vi "map_diag_stiffback.vi"() -> ()   [LabVIEW 2015]
panel:
  in  "Done ?":bool
  out "Mapping DX ext":string
  out "Mapping SX ext":string
  out "Mapping DX int":string
  out "Mapping SX int":string
  in  "z inizio":bool
  in  "x piastra":bool
  in  "z piastra":bool
  in  "Done":bool
  in  "y inizio":bool
  in  "Positioning Done":bool
  in  "x inizio":bool
  in  "y inizio":bool
  in  "Positioning Done":bool
  in  "y inizio":bool
  in  "Positioning Done":bool
  in  "KILL":bool
  in  "PAUSE":bool
  in  "RESUME":bool
  in  "QUIT":bool
  in  "Positioning Done":bool
  in  "y inizio":bool
  in  "x inizio":bool
  in  "End":bool
  in  "zero z - end":bool
  in  "zero x - end":bool
  in  "zero y - end":bool
  out "output":string
  out "command":string
  in  "zero done":bool
  in  "zero z":bool
  in  "zero x":bool
  in  "zero y":bool
  # "Posiziono in zero"
  # "Comandi di emergenza"
  # "Vado al punto di \nazzeramento"
  # "Vado al punto di partenza\nDiagonale Left Internal"
  # "Vado al punto di partenza\nDiagonale Right Internal"
  # "Vado al punto di partenza\nDiagonale Left External"
  # "Vado al punto di partenza\nDiagonale Right External"
  # "Ritorno a zero"
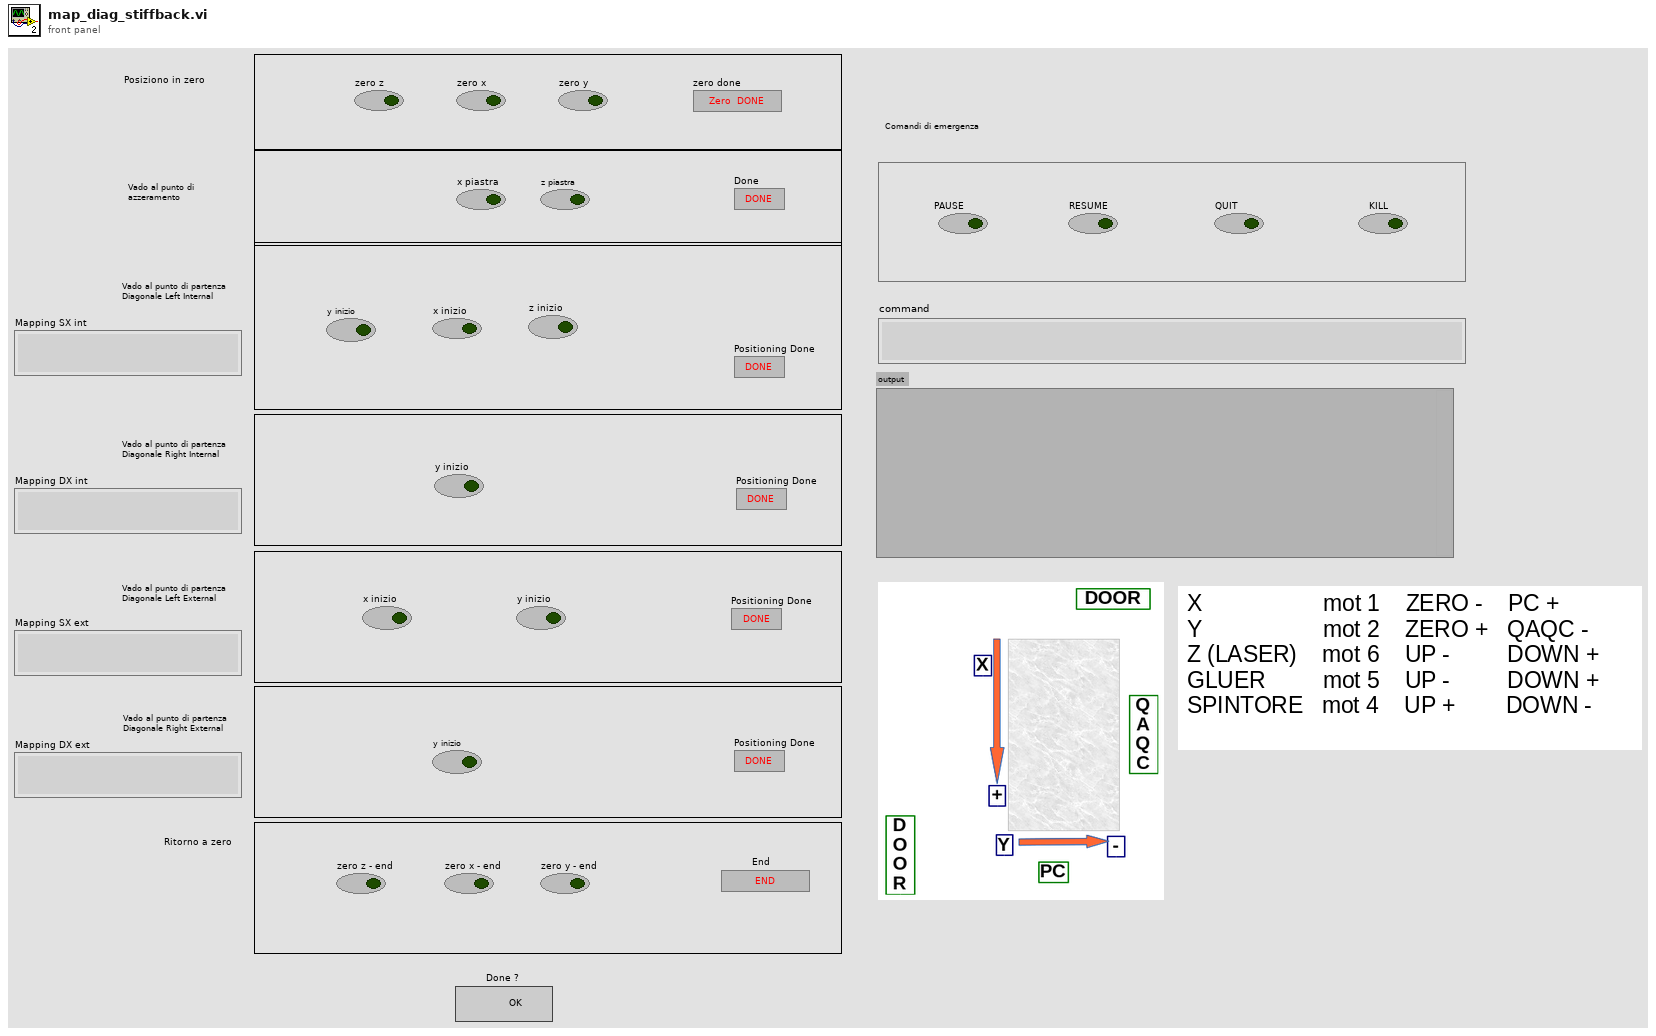
[diagram p1: front panel]
types:
  T1 = enum16{"open", "replace", "create", "open or create", "replace or create", "replace or create with confirmation"}
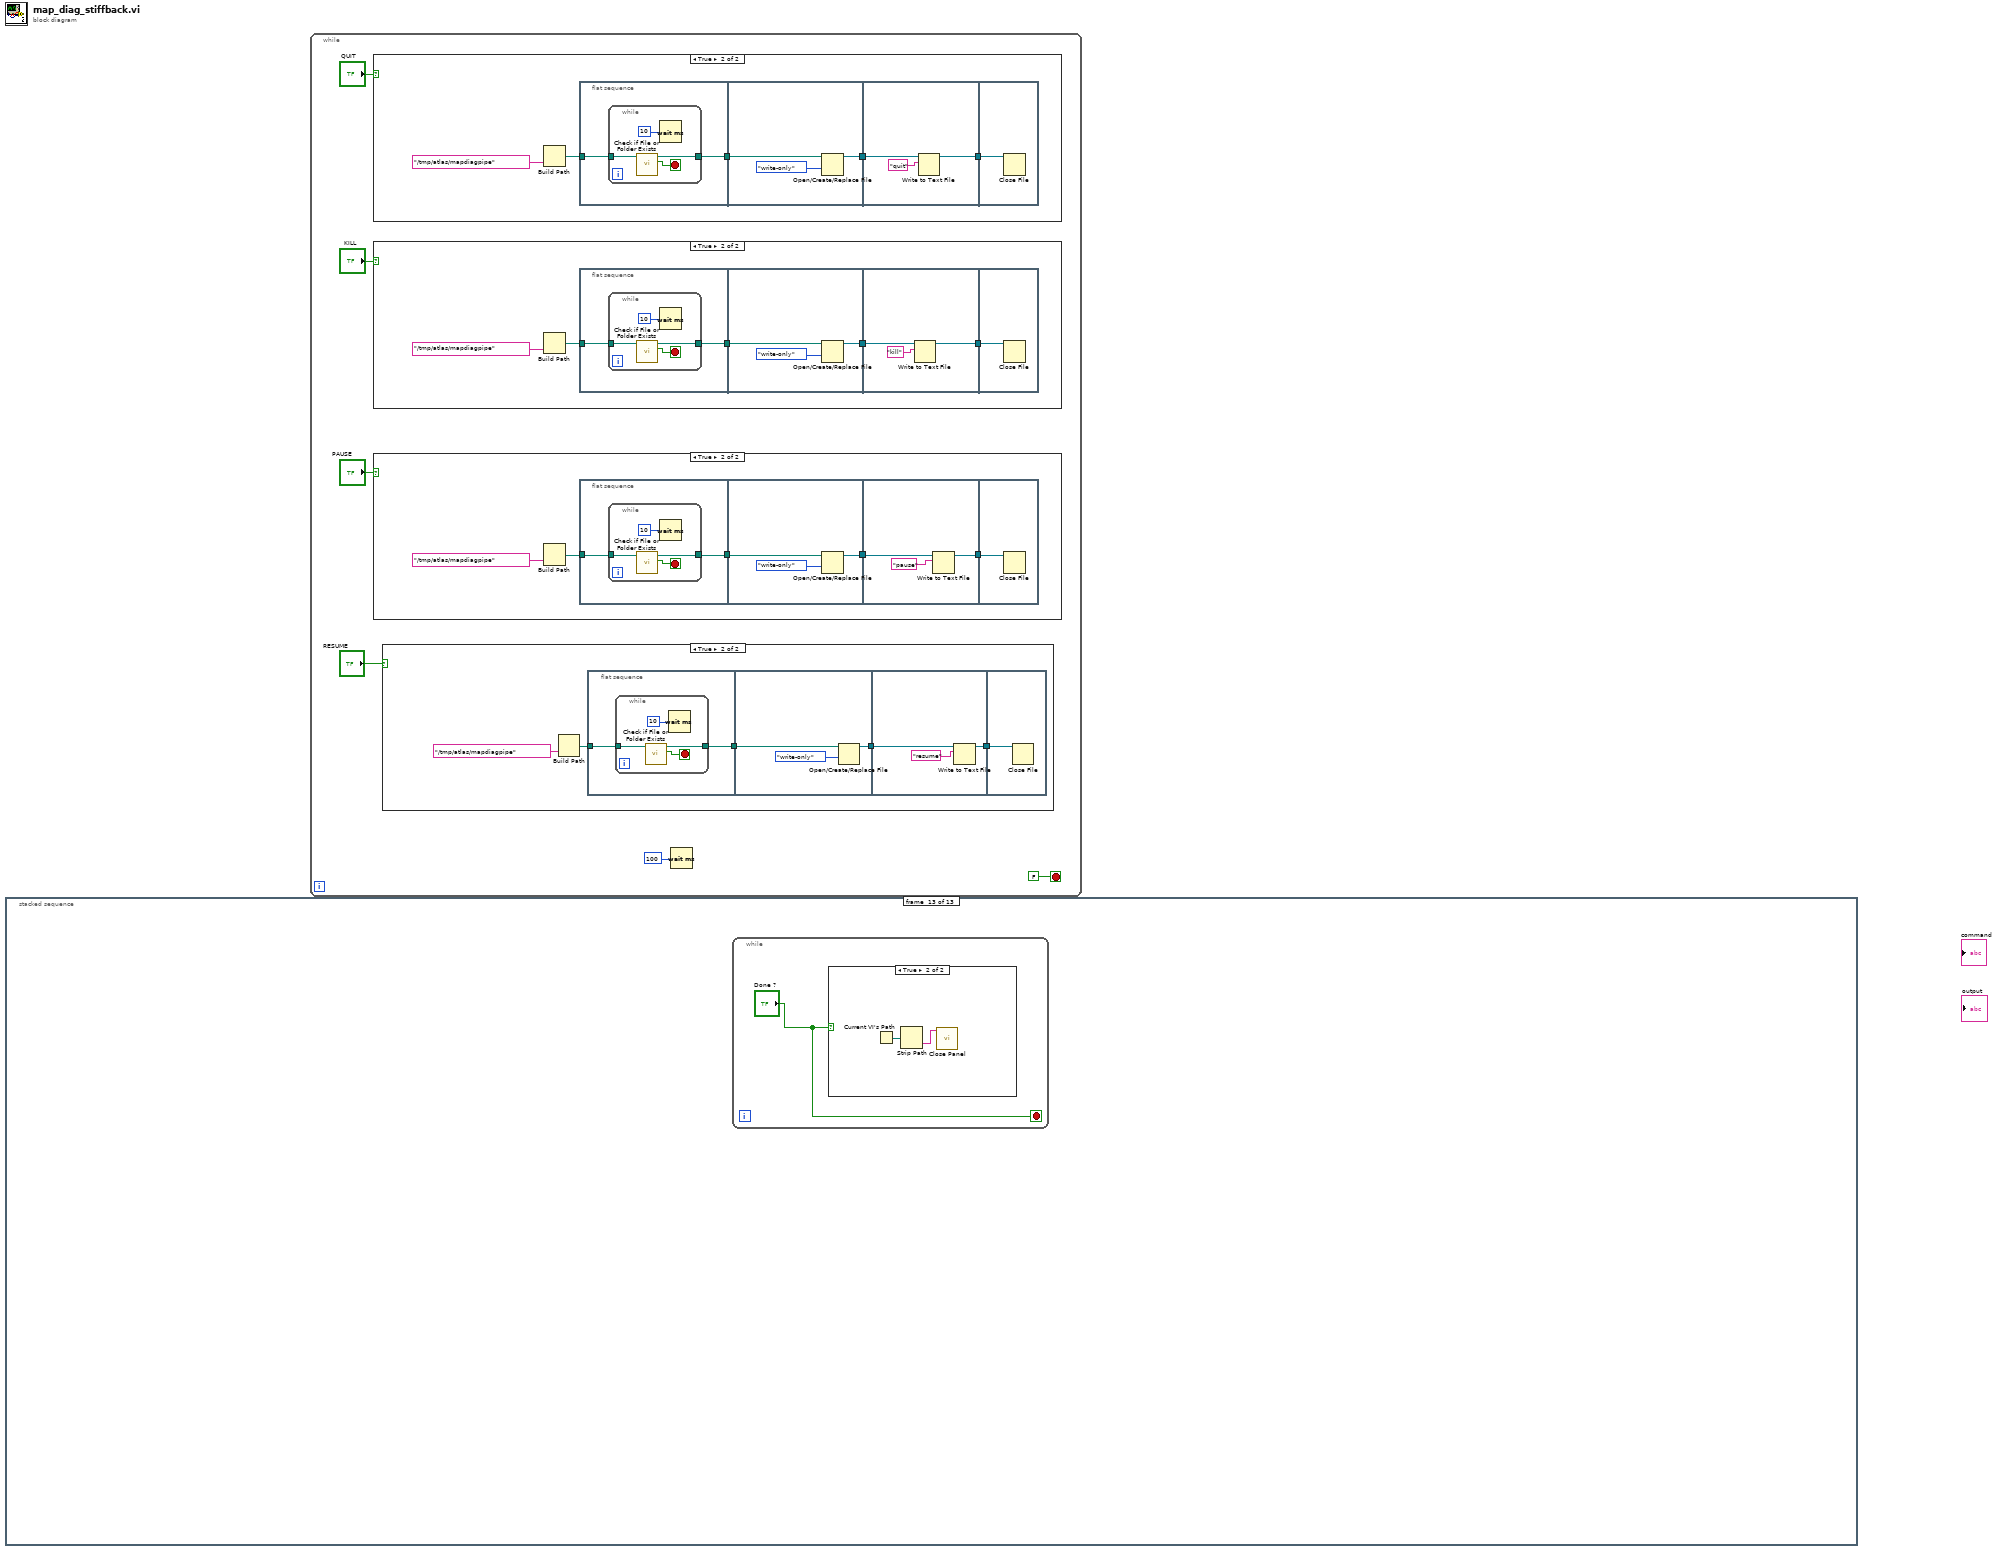
[diagram p0: block diagram]
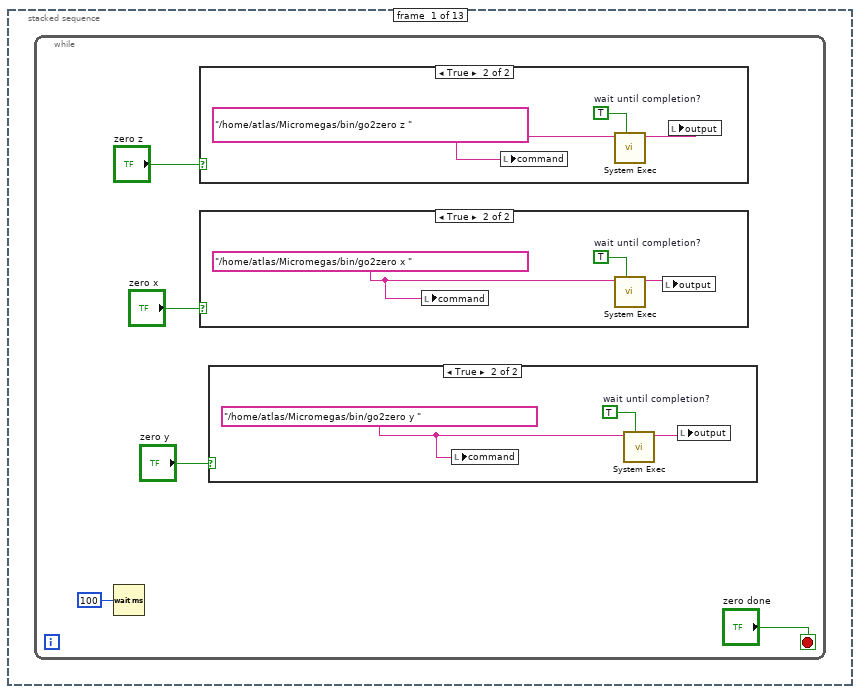
[diagram p6: hidden frame]
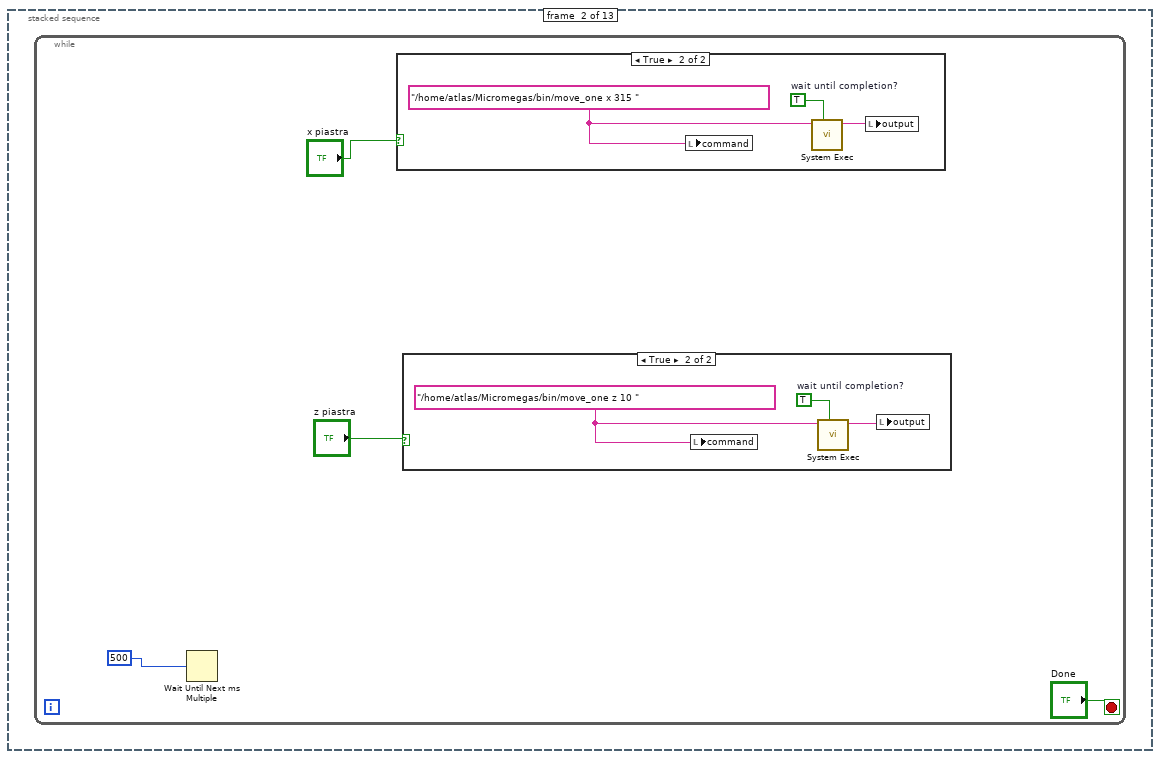
[diagram p10: hidden frame]
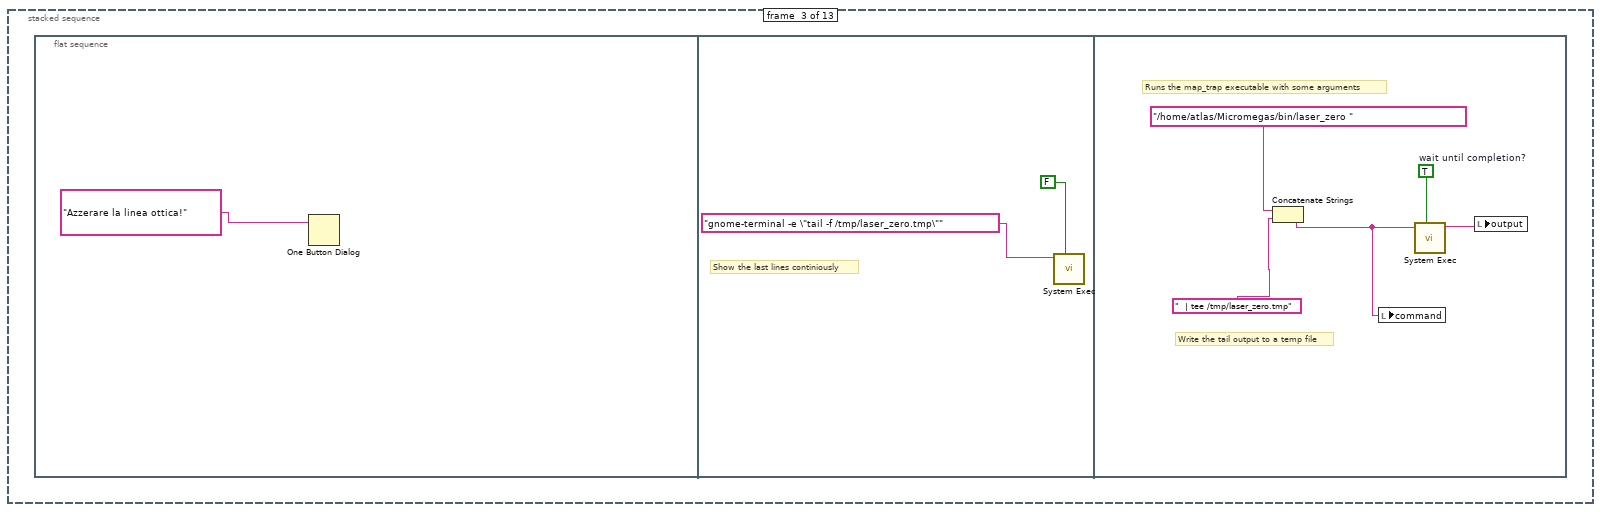
[diagram p13: hidden frame]
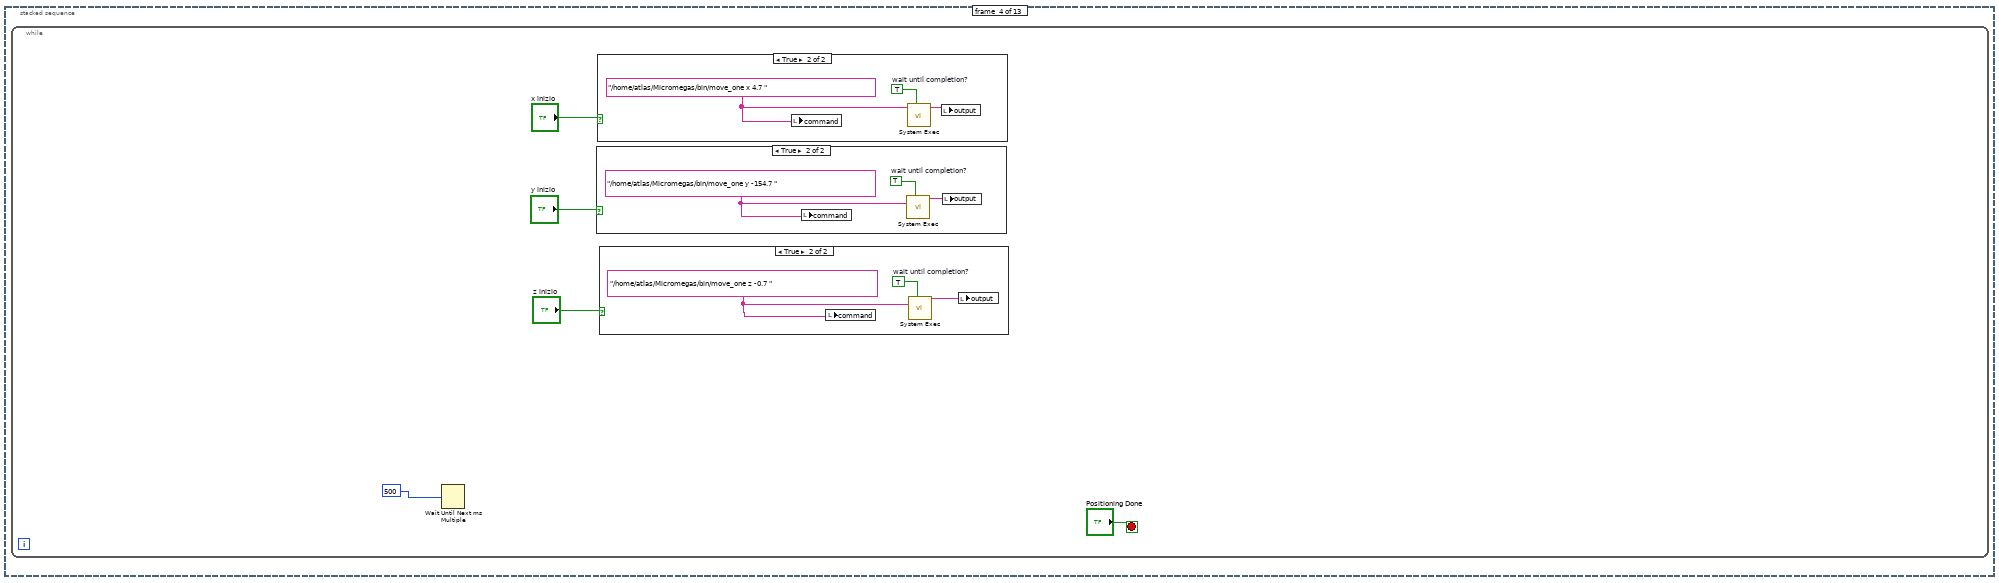
[diagram p14: hidden frame]
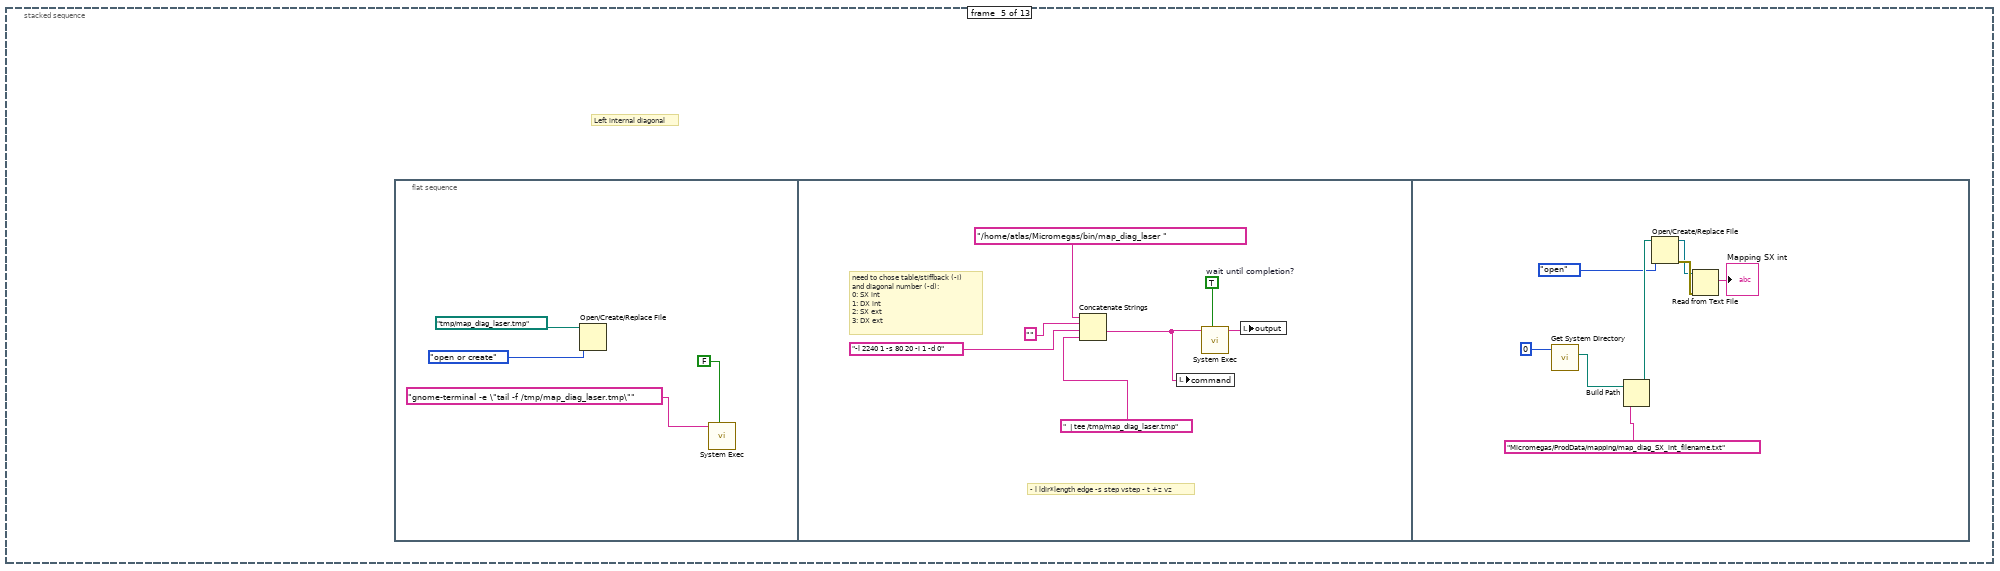
[diagram p18: hidden frame]
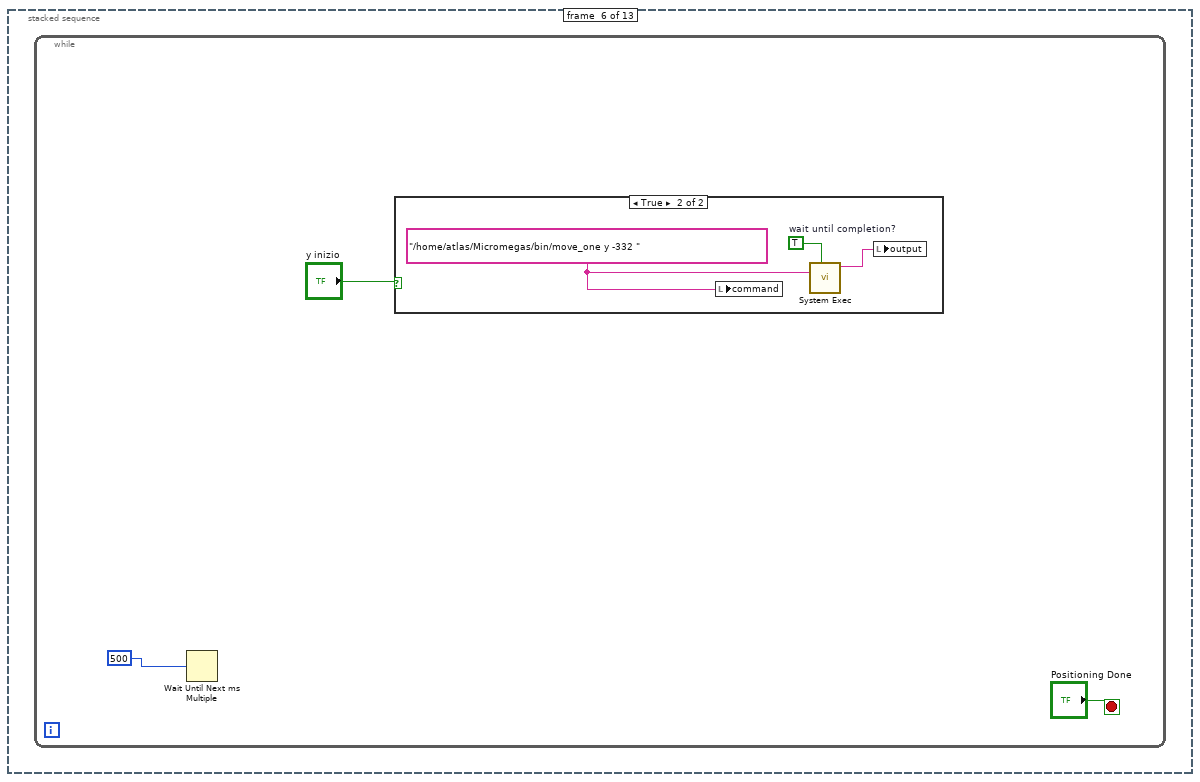
[diagram p19: hidden frame]
diagram:
  n1 = stacked-sequence {
    frame #0 {
      n2 = while {
        stop <- "zero done" stop-if-true
        n3 = Wait (ms)(milliseconds to wait=u32 100) -> ()  [unwired: 1 out]
        n4 = case shown="True" "zero z" {
          frame False {
          }
          frame True {
            w13 = "/home/atlas/Micromegas/bin/go2zero z " ("string")
            w14 = TRUE  # wait until completion?
            n5 = local write "command"(w13) -> ()
            n6 = call <vilib>:"System Exec.vi"("wait until completion? (T)"=w14, "command line"=w13) -> ("standard output"=w12:string)  [unwired: 6 in, 3 out]
            n7 = local write "output"(w12) -> ()
          }
        }
        n8 = case shown="True" "zero x" {
          frame False {
          }
          frame True {
            w10 = "/home/atlas/Micromegas/bin/go2zero x " ("string")
            w11 = TRUE  # wait until completion?
            n9 = local write "command"(w10) -> ()
            n10 = call <vilib>:"System Exec.vi"("wait until completion? (T)"=w11, "command line"=w10) -> ("standard output"=w9:string)  [unwired: 6 in, 3 out]
            n11 = local write "output"(w9) -> ()
          }
        }
        n12 = case shown="True" "zero y" {
          frame False {
          }
          frame True {
            w7 = "/home/atlas/Micromegas/bin/go2zero y " ("string")
            w8 = TRUE  # wait until completion?
            n13 = local write "command"(w7) -> ()
            n14 = call <vilib>:"System Exec.vi"("wait until completion? (T)"=w8, "command line"=w7) -> ("standard output"=w6:string)  [unwired: 6 in, 3 out]
            n15 = local write "output"(w6) -> ()
          }
        }
      }
    }
    frame #1 {
      n16 = while {
        stop <- "Done" stop-if-true
        n17 = Wait Until Next ms Multiple(millisecond multiple=u32 500 ("millisecond timer value")) -> ()  [unwired: 1 out]
        n18 = case shown="True" "x piastra" {
          frame False {
          }
          frame True {
            w22 = "/home/atlas/Micromegas/bin/move_one x 315 " ("string")
            w24 = TRUE  # wait until completion?
            n19 = local write "command"(w22) -> ()
            n20 = call <vilib>:"System Exec.vi"("wait until completion? (T)"=w24, "command line"=w22) -> ("standard output"=w23:string)  [unwired: 6 in, 3 out]
            n21 = local write "output"(w23) -> ()
          }
        }
        n22 = case shown="True" "z piastra" {
          frame False {
          }
          frame True {
            w20 = "/home/atlas/Micromegas/bin/move_one z 10 " ("string")
            w21 = TRUE  # wait until completion?
            n23 = local write "command"(w20) -> ()
            n24 = call <vilib>:"System Exec.vi"("wait until completion? (T)"=w21, "command line"=w20) -> ("standard output"=w19:string)  [unwired: 6 in, 3 out]
            n25 = local write "output"(w19) -> ()
          }
        }
      }
    }
    frame #2 {
      n26 = flat-sequence {
        frame #0 {
          n27 = One Button Dialog(message="Azzerare la linea ottica!") -> ()  [unwired: 1 in, 1 out]
        }
        frame #1 {
          # "Show the last lines continiously"
          n28 = call <vilib>:"System Exec.vi"("wait until completion? (T)"=FALSE, "command line"="gnome-terminal -e \"tail -f /tmp/laser_zero.tmp\"") -> ()  [unwired: 6 in, 4 out]
        }
        frame #2 {
          w32 = TRUE  # wait until completion?
          # "Write the tail output to a temp file"
          # "Runs the map_trap executable with some arguments"
          n29 = Concatenate Strings("/home/atlas/Micromegas/bin/laser_zero " ("string"), "  | tee /tmp/laser_zero.tmp" ("string")) -> (w28:string)
          n30 = local write "command"(w28) -> ()
          n31 = call <vilib>:"System Exec.vi"("wait until completion? (T)"=w32, "command line"=w28) -> ("standard output"=w29:string)  [unwired: 6 in, 3 out]
          n32 = local write "output"(w29) -> ()
        }
      }
    }
    frame #3 {
      n33 = while {
        stop <- "Positioning Done" stop-if-true
        n34 = Wait Until Next ms Multiple(millisecond multiple=u32 500 ("millisecond timer value")) -> ()  [unwired: 1 out]
        n35 = case shown="True" "y inizio" {
          frame False {
          }
          frame True {
            w41 = "/home/atlas/Micromegas/bin/move_one y -154.7 " ("string")
            w43 = TRUE  # wait until completion?
            n36 = local write "command"(w41) -> ()
            n37 = call <vilib>:"System Exec.vi"("wait until completion? (T)"=w43, "command line"=w41) -> ("standard output"=w42:string)  [unwired: 6 in, 3 out]
            n38 = local write "output"(w42) -> ()
          }
        }
        n39 = case shown="True" "x inizio" {
          frame False {
          }
          frame True {
            w44 = "/home/atlas/Micromegas/bin/move_one x 4.7 " ("string")
            w46 = TRUE  # wait until completion?
            n40 = local write "command"(w44) -> ()
            n41 = call <vilib>:"System Exec.vi"("wait until completion? (T)"=w46, "command line"=w44) -> ("standard output"=w45:string)  [unwired: 6 in, 3 out]
            n42 = local write "output"(w45) -> ()
          }
        }
        n43 = case shown="True" "z inizio" {
          frame False {
          }
          frame True {
            w38 = "/home/atlas/Micromegas/bin/move_one z -0.7 " ("string")
            w40 = TRUE  # wait until completion?
            n44 = local write "command"(w38) -> ()
            n45 = call <vilib>:"System Exec.vi"("wait until completion? (T)"=w40, "command line"=w38) -> ("standard output"=w39:string)  [unwired: 6 in, 3 out]
            n46 = local write "output"(w39) -> ()
          }
        }
      }
    }
    frame #4 {
      # "Left internal diagonal"
      n47 = flat-sequence {
        frame #0 {
          n48 = Open/Create/Replace File(file path (use dialog)=path "/tmp/map_diag_laser.tmp", operation (0:open)=T1."open or create") -> ()  [unwired: 4 in, 3 out]
          n49 = call <vilib>:"System Exec.vi"("wait until completion? (T)"=FALSE, "command line"="gnome-terminal -e \"tail -f /tmp/map_diag_laser.tmp\"") -> ()  [unwired: 6 in, 4 out]
        }
        frame #1 {
          w57 = TRUE  # wait until completion?
          # "need to chose table/stiffback (-i)\nand diagonal number (-d):\n0: SX int\n1: DX int\n2: SX ext\n3: DX ext"
          # "- l ldir*length edge -s step vstep - t +z vz"
          n50 = Concatenate Strings("/home/atlas/Micromegas/bin/map_diag_laser " ("string"), "" ("string"), "-l 2240 1 -s 80 20 -i 1 -d 0" ("string"), "  | tee /tmp/map_diag_laser.tmp" ("string")) -> (w54:string)
          n51 = local write "command"(w54) -> ()
          n52 = call <vilib>:"System Exec.vi"("wait until completion? (T)"=w57, "command line"=w54) -> ("standard output"=w55:string)  [unwired: 6 in, 3 out]
          n53 = local write "output"(w55) -> ()
        }
        frame #2 {
          n54 = call <vilib>:"Get System Directory.vi"("system directory type"=0) -> ("system directory"=w64:path)  [unwired: 10 in]
          n55 = Build Path(base path=w64, name or relative path="Micromegas/ProdData/mapping/map_diag_SX_int_filename.txt") -> (appended path=w65:path)
          n56 = Open/Create/Replace File(file path (use dialog)=w65, operation (0:open)=T1."open") -> (refnum out=w59:refnum<file>, error out=w60:errorcluster)  [unwired: 4 in, 1 out]
          n57 = Read from Text File(file (use dialog)=w59, error in=w60) -> (text=→"Mapping SX int":string)  [unwired: 2 in, 3 out]
        }
      }
    }
    frame #5 {
      n58 = while {
        stop <- "Positioning Done" stop-if-true
        n59 = Wait Until Next ms Multiple(millisecond multiple=u32 500 ("millisecond timer value")) -> ()  [unwired: 1 out]
        n60 = case shown="True" "y inizio" {
          frame False {
          }
          frame True {
            w69 = "/home/atlas/Micromegas/bin/move_one y -332 " ("string")
            w71 = TRUE  # wait until completion?
            n61 = local write "command"(w69) -> ()
            n62 = call <vilib>:"System Exec.vi"("wait until completion? (T)"=w71, "command line"=w69) -> ("standard output"=w70:string)  [unwired: 6 in, 3 out]
            n63 = local write "output"(w70) -> ()
          }
        }
      }
    }
    frame #6 {
      n64 = flat-sequence {
        frame #0 {
          w78 = TRUE  # wait until completion?
          # "need to chose table/stiffback (-i)\nand diagonal number (-d):\n0: SX int\n1: DX int\n2: SX ext\n3: DX ext"
          # "Right internal diagonal"
          # "- l ldir*length edge -s step vstep - t +z vz"
          n65 = Concatenate Strings("/home/atlas/Micromegas/bin/map_diag_laser " ("string"), "" ("string"), "-l -2240 0 -s 80 20 -i 1 -d 1" ("string"), "  | tee /tmp/map_diag_laser.tmp" ("string")) -> (w72:string)
          n66 = call <vilib>:"System Exec.vi"("wait until completion? (T)"=w78, "command line"=w72) -> ("standard output"=w73:string)  [unwired: 6 in, 3 out]
          n67 = local write "command"(w72) -> ()
          n68 = local write "output"(w73) -> ()
        }
        frame #1 {
          n69 = call <vilib>:"Get System Directory.vi"("system directory type"=0) -> ("system directory"=w85:path)  [unwired: 10 in]
          n70 = Build Path(base path=w85, name or relative path="Micromegas/ProdData/mapping/map_diag_DX_int_filename.txt") -> (appended path=w86:path)
          n71 = Open/Create/Replace File(file path (use dialog)=w86, operation (0:open)=T1."open") -> (refnum out=w80:refnum<file>, error out=w81:errorcluster)  [unwired: 4 in, 1 out]
          n72 = Read from Text File(file (use dialog)=w80, error in=w81) -> (text=→"Mapping DX int":string)  [unwired: 2 in, 3 out]
        }
      }
    }
    frame #7 {
      n73 = while {
        stop <- "Positioning Done" stop-if-true
        n74 = Wait Until Next ms Multiple(millisecond multiple=u32 500 ("millisecond timer value")) -> ()  [unwired: 1 out]
        n75 = case shown="True" "x inizio" {
          frame False {
          }
          frame True {
            w91 = "/home/atlas/Micromegas/bin/move_one x 11 " ("string")
            w93 = TRUE  # wait until completion?
            n76 = local write "command"(w91) -> ()
            n77 = call <vilib>:"System Exec.vi"("wait until completion? (T)"=w93, "command line"=w91) -> ("standard output"=w92:string)  [unwired: 6 in, 3 out]
            n78 = local write "output"(w92) -> ()
          }
        }
        n79 = case shown="True" "y inizio" {
          frame False {
          }
          frame True {
            w94 = "/home/atlas/Micromegas/bin/move_one y 1190 " ("string")
            w96 = TRUE  # wait until completion?
            n80 = local write "command"(w94) -> ()
            n81 = call <vilib>:"System Exec.vi"("wait until completion? (T)"=w96, "command line"=w94) -> ("standard output"=w95:string)  [unwired: 6 in, 3 out]
            n82 = local write "output"(w95) -> ()
          }
        }
      }
    }
    frame #8 {
      n83 = flat-sequence {
        frame #0 {
          w103 = TRUE  # wait until completion?
          # "need to chose table/stiffback (-i)\nand diagonal number (-d):\n0: SX int\n1: DX int\n2: SX ext\n3: DX ext"
          # "Left external diagonal"
          # "- l ldir*length edge -s step vstep - t +z vz"
          n84 = Concatenate Strings("/home/atlas/Micromegas/bin/map_diag_laser " ("string"), "" ("string"), "-l 2200 1 -s 110 20 -i 1 -d 2" ("string"), "  | tee /tmp/map_diag_laser.tmp" ("string")) -> (w97:string)
          n85 = call <vilib>:"System Exec.vi"("wait until completion? (T)"=w103, "command line"=w97) -> ("standard output"=w98:string)  [unwired: 6 in, 3 out]
          n86 = local write "command"(w97) -> ()
          n87 = local write "output"(w98) -> ()
        }
        frame #1 {
          n88 = call <vilib>:"Get System Directory.vi"("system directory type"=0) -> ("system directory"=w110:path)  [unwired: 10 in]
          n89 = Build Path(base path=w110, name or relative path="Micromegas/ProdData/mapping/map_diag_SX_ext_filename.txt") -> (appended path=w111:path)
          n90 = Open/Create/Replace File(file path (use dialog)=w111, operation (0:open)=T1."open") -> (refnum out=w105:refnum<file>, error out=w106:errorcluster)  [unwired: 4 in, 1 out]
          n91 = Read from Text File(file (use dialog)=w105, error in=w106) -> (text=→"Mapping SX ext":string)  [unwired: 2 in, 3 out]
        }
      }
    }
    frame #9 {
      n92 = while {
        stop <- "Positioning Done" stop-if-true
        n93 = Wait Until Next ms Multiple(millisecond multiple=u32 500 ("millisecond timer value")) -> ()  [unwired: 1 out]
        n94 = case shown="True" "y inizio" {
          frame False {
          }
          frame True {
            w115 = "/home/atlas/Micromegas/bin/move_one y -505 " ("string")
            w117 = TRUE  # wait until completion?
            n95 = local write "command"(w115) -> ()
            n96 = call <vilib>:"System Exec.vi"("wait until completion? (T)"=w117, "command line"=w115) -> ("standard output"=w116:string)  [unwired: 6 in, 3 out]
            n97 = local write "output"(w116) -> ()
          }
        }
      }
    }
    frame #10 {
      n98 = flat-sequence {
        frame #0 {
          w124 = TRUE  # wait until completion?
          # "need to chose table/stiffback (-i)\nand diagonal number (-d):\n0: SX int\n1: DX int\n2: SX ext\n3: DX ext"
          # "Right external diagonal"
          # "- l ldir*length edge -s step vstep - t +z vz"
          n99 = Concatenate Strings("/home/atlas/Micromegas/bin/map_diag_laser " ("string"), "" ("string"), "-l -2200 0 -s 110 20 -i 1 -d 3" ("string"), "  | tee /tmp/map_diag_laser.tmp" ("string")) -> (w118:string)
          n100 = call <vilib>:"System Exec.vi"("wait until completion? (T)"=w124, "command line"=w118) -> ("standard output"=w119:string)  [unwired: 6 in, 3 out]
          n101 = local write "command"(w118) -> ()
          n102 = local write "output"(w119) -> ()
        }
        frame #1 {
          n103 = call <vilib>:"Get System Directory.vi"("system directory type"=0) -> ("system directory"=w131:path)  [unwired: 10 in]
          n104 = Build Path(base path=w131, name or relative path="Micromegas/ProdData/mapping/map_diag_DX_ext_filename.txt") -> (appended path=w132:path)
          n105 = Open/Create/Replace File(file path (use dialog)=w132, operation (0:open)=T1."open") -> (refnum out=w126:refnum<file>, error out=w127:errorcluster)  [unwired: 4 in, 1 out]
          n106 = Read from Text File(file (use dialog)=w126, error in=w127) -> (text=→"Mapping DX ext":string)  [unwired: 2 in, 3 out]
        }
      }
    }
    frame #11 {
      n107 = while {
        stop <- "End" stop-if-true
        n108 = Wait (ms)(milliseconds to wait=u32 100) -> ()  [unwired: 1 out]
        n109 = case shown="True" "zero z - end" {
          frame False {
          }
          frame True {
            w145 = "/home/atlas/Micromegas/bin/go2zero z " ("string")
            w146 = TRUE  # wait until completion?
            n110 = local write "command"(w145) -> ()
            n111 = call <vilib>:"System Exec.vi"("wait until completion? (T)"=w146, "command line"=w145) -> ("standard output"=w144:string)  [unwired: 6 in, 3 out]
            n112 = local write "output"(w144) -> ()
          }
        }
        n113 = case shown="True" "zero x - end" {
          frame False {
          }
          frame True {
            w142 = "/home/atlas/Micromegas/bin/go2zero x " ("string")
            w143 = TRUE  # wait until completion?
            n114 = local write "command"(w142) -> ()
            n115 = call <vilib>:"System Exec.vi"("wait until completion? (T)"=w143, "command line"=w142) -> ("standard output"=w141:string)  [unwired: 6 in, 3 out]
            n116 = local write "output"(w141) -> ()
          }
        }
        n117 = case shown="True" "zero y - end" {
          frame False {
          }
          frame True {
            w139 = "/home/atlas/Micromegas/bin/go2zero y " ("string")
            w140 = TRUE  # wait until completion?
            n118 = local write "command"(w139) -> ()
            n119 = call <vilib>:"System Exec.vi"("wait until completion? (T)"=w140, "command line"=w139) -> ("standard output"=w138:string)  [unwired: 6 in, 3 out]
            n120 = local write "output"(w138) -> ()
          }
        }
      }
    }
    frame #12 {
      n121 = while {
        stop <- "Done ?" stop-if-true
        n122 = case shown="True" "Done ?" {
          frame False {
          }
          frame True {
            n123 = Current VI's Path() -> (path=w148:path)
            n124 = Strip Path(path=w148) -> (name=w149:string)  [unwired: 1 out]
            n125 = call <vilib>:"Close Panel.vi"("VI name"=w149) -> ()  [unwired: 10 in, 1 out]
          }
        }
      }
    }
  }
  n126 = while {
    stop <- FALSE stop-if-true
    n127 = case shown="True" "QUIT" {
      frame False {
      }
      frame True {
        n128 = Build Path(name or relative path="/tmp/atlas/mapdiagpipe" ("string")) -> (appended path=w210:path)  [unwired: 1 in]
        n129 = flat-sequence {
          tunnel: [w216] -> w214
          tunnel: w210 -> [w215]
          tunnel: w214 -> [w223]
          tunnel: [w221] -> w213
          tunnel: w213 -> [w226]
          tunnel: [w225] -> w212
          tunnel: w212 -> [w227]
          frame #0 {
            n130 = while {
              tunnel: [w218] -> w216
              tunnel: w215 -> [w217]
              stop <- w219 stop-if-true
              n131 = call <vilib>:"Check if File or Folder Exists.vi"("path"=w217) -> ("file or folder exists?"=w219:bool, "dup path"=w218:path)  [unwired: 8 in, 1 out]
              n132 = Wait (ms)(milliseconds to wait=u32 10) -> ()  [unwired: 1 out]
            }
          }
          frame #1 {
            n133 = Open/Create/Replace File(file path (use dialog)=w223, access (0:read/write)=enum16{"read/write", "read-only", "write-only"}."write-only") -> (refnum out=w221:refnum<file>)  [unwired: 4 in, 2 out]
          }
          frame #2 {
            n134 = Write to Text File(file (use dialog)=w226, text="quit") -> (refnum out=w225:refnum<file>)  [unwired: 2 in, 2 out]
          }
          frame #3 {
            n135 = Close File(refnum=w227) -> ()  [unwired: 1 in, 2 out]
          }
        }
      }
    }
    n136 = case shown="True" "KILL" {
      frame False {
      }
      frame True {
        n137 = Build Path(name or relative path="/tmp/atlas/mapdiagpipe" ("string")) -> (appended path=w174:path)  [unwired: 1 in]
        n138 = flat-sequence {
          tunnel: [w180] -> w178
          tunnel: w174 -> [w179]
          tunnel: w178 -> [w187]
          tunnel: [w185] -> w177
          tunnel: w177 -> [w190]
          tunnel: [w189] -> w176
          tunnel: w176 -> [w191]
          frame #0 {
            n139 = while {
              tunnel: [w182] -> w180
              tunnel: w179 -> [w181]
              stop <- w183 stop-if-true
              n140 = call <vilib>:"Check if File or Folder Exists.vi"("path"=w181) -> ("file or folder exists?"=w183:bool, "dup path"=w182:path)  [unwired: 8 in, 1 out]
              n141 = Wait (ms)(milliseconds to wait=u32 10) -> ()  [unwired: 1 out]
            }
          }
          frame #1 {
            n142 = Open/Create/Replace File(file path (use dialog)=w187, access (0:read/write)=enum16{"read/write", "read-only", "write-only"}."write-only") -> (refnum out=w185:refnum<file>)  [unwired: 4 in, 2 out]
          }
          frame #2 {
            n143 = Write to Text File(file (use dialog)=w190, text="kill") -> (refnum out=w189:refnum<file>)  [unwired: 2 in, 2 out]
          }
          frame #3 {
            n144 = Close File(refnum=w191) -> ()  [unwired: 1 in, 2 out]
          }
        }
      }
    }
    n145 = case shown="True" "PAUSE" {
      frame False {
      }
      frame True {
        n146 = Build Path(name or relative path="/tmp/atlas/mapdiagpipe" ("string")) -> (appended path=w156:path)  [unwired: 1 in]
        n147 = flat-sequence {
          tunnel: [w162] -> w160
          tunnel: w156 -> [w161]
          tunnel: w160 -> [w169]
          tunnel: [w167] -> w159
          tunnel: w159 -> [w172]
          tunnel: [w171] -> w158
          tunnel: w158 -> [w173]
          frame #0 {
            n148 = while {
              tunnel: [w164] -> w162
              tunnel: w161 -> [w163]
              stop <- w165 stop-if-true
              n149 = call <vilib>:"Check if File or Folder Exists.vi"("path"=w163) -> ("file or folder exists?"=w165:bool, "dup path"=w164:path)  [unwired: 8 in, 1 out]
              n150 = Wait (ms)(milliseconds to wait=u32 10) -> ()  [unwired: 1 out]
            }
          }
          frame #1 {
            n151 = Open/Create/Replace File(file path (use dialog)=w169, access (0:read/write)=enum16{"read/write", "read-only", "write-only"}."write-only") -> (refnum out=w167:refnum<file>)  [unwired: 4 in, 2 out]
          }
          frame #2 {
            n152 = Write to Text File(file (use dialog)=w172, text="pause") -> (refnum out=w171:refnum<file>)  [unwired: 2 in, 2 out]
          }
          frame #3 {
            n153 = Close File(refnum=w173) -> ()  [unwired: 1 in, 2 out]
          }
        }
      }
    }
    n154 = case shown="True" "RESUME" {
      frame False {
      }
      frame True {
        n155 = Build Path(name or relative path="/tmp/atlas/mapdiagpipe" ("string")) -> (appended path=w192:path)  [unwired: 1 in]
        n156 = flat-sequence {
          tunnel: [w198] -> w196
          tunnel: w192 -> [w197]
          tunnel: w196 -> [w205]
          tunnel: [w203] -> w195
          tunnel: w195 -> [w208]
          tunnel: [w207] -> w194
          tunnel: w194 -> [w209]
          frame #0 {
            n157 = while {
              tunnel: [w200] -> w198
              tunnel: w197 -> [w199]
              stop <- w201 stop-if-true
              n158 = call <vilib>:"Check if File or Folder Exists.vi"("path"=w199) -> ("file or folder exists?"=w201:bool, "dup path"=w200:path)  [unwired: 8 in, 1 out]
              n159 = Wait (ms)(milliseconds to wait=u32 10) -> ()  [unwired: 1 out]
            }
          }
          frame #1 {
            n160 = Open/Create/Replace File(file path (use dialog)=w205, access (0:read/write)=enum16{"read/write", "read-only", "write-only"}."write-only") -> (refnum out=w203:refnum<file>)  [unwired: 4 in, 2 out]
          }
          frame #2 {
            n161 = Write to Text File(file (use dialog)=w208, text="resume") -> (refnum out=w207:refnum<file>)  [unwired: 2 in, 2 out]
          }
          frame #3 {
            n162 = Close File(refnum=w209) -> ()  [unwired: 1 in, 2 out]
          }
        }
      }
    }
    n163 = Wait (ms)(milliseconds to wait=100) -> ()  [unwired: 1 out]
  }
